vi "init.vi"(0 "SM_CW High Test in":refnum<class "SM_CW High Test.lvclass">, 5 "ILC":refnum<class "ILC.lvclass">, 7 "ILC Digital Output Test":T1, 9 "Log":refnum<class "ITestLog.lvclass">, 11 "error in (no error)":errorcluster) -> (4 "SM_CW High Test out":refnum<class "SM_CW High Test.lvclass">, 15 "error out":errorcluster)   [LabVIEW 2015, in "SM_CW High Test.lvclass"]
uses:
  SM_CW High Test.lvclass
  <userlib>/Common/ILC/ILC/ILC.lvclass
  Typedefs/ILC Digital Output Test.ctl
  Typedefs/Digital Signal Level.ctl
  Model/TestLog/ITestLog/ITestLog.lvclass
  SM_CW High Test.lvclass/SM_CW High Test.ctl
  Typedefs/ILCBTTypedefs.lvlib
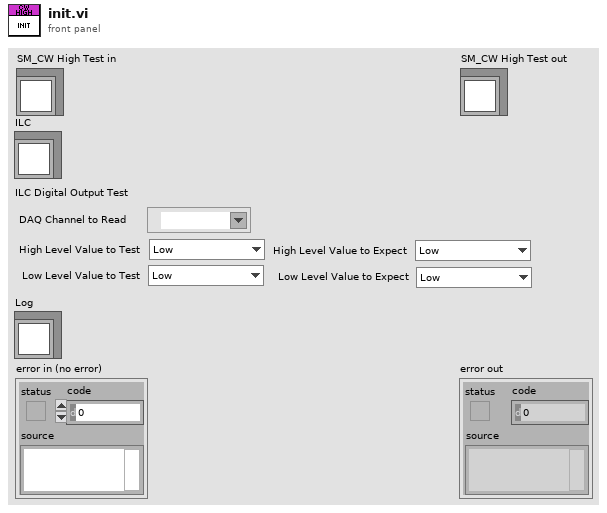
[diagram p1: front panel]
types:
  T1 = typedef "ILCBTTypedefs.lvlib/ILC Digital Output Test.ctl" = cluster{"DAQ Channel to Read":refnum<k21>, "High Level Value to Test":T2, "High Level Value to Expect":T2, "Low Level Value to Test":T2, "Low Level Value to Expect":T2}
  T2 = typedef "ILCBTTypedefs.lvlib/Digital Signal Level.ctl" = enum16{"Low", "High"}
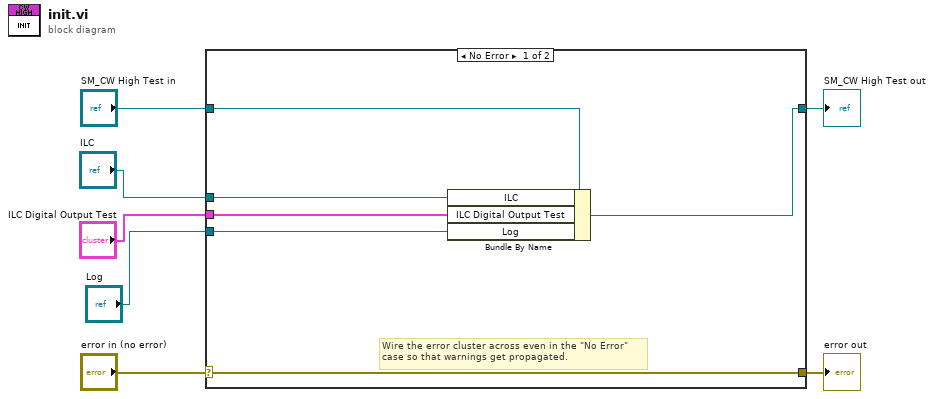
[diagram p0: block diagram]
diagram:
  n1 = case shown="No Error" "error in (no error)" {
    selector: "error in (no error)" -> [w13 w15]
    tunnel: [w13 w15] -> w6
    tunnel: [w11 w14] -> w4
    tunnel: "SM_CW High Test in" -> [w12 w14]
    tunnel: "ILC" -> [w10 _]
    tunnel: "ILC Digital Output Test" -> [w9 _]
    tunnel: "Log" -> [w8 _]
    frame No Error {
      # "Wire the error cluster across even in the \"No Error\"\ncase so that warnings get propagated."
      n2 = Bundle By Name(cluster=w12, "ILC"=w10, "ILC Digital Output Test"=w9, "Log"=w8) -> (w11:refnum<class "SM_CW High Test.lvclass">)
    }
    frame Error {
    }
  }
  "error out" <- w6
  "SM_CW High Test out" <- w4
